vi "Read Device Identification.vi"(8 "error in (no error)":errorcluster, 9 "object ID":u8, 10 "device ID category":T1(ring), 11 "Modbus master in":refnum<class "Modbus Master.lvclass">) -> (0 "error out":errorcluster, 2 "objects":cluster{"object ID":u8, "value":string}[](array[cluster]) {"object ID" format="%x"}, 3 "Modbus master out":refnum<class "Modbus Master.lvclass">)   [LabVIEW 2017, in "Modbus Master.lvclass"]
doc: "Returns the device identification of a Modbus slave. Device identification consists of data elements called objects. Each object has an identification number and stores Modbus slave information."
uses:
  <vilib>/Modbus/master/Modbus Master.lvclass
  C:/builds/penguin/iak/lvdsc/trunk/17.0/lv/vi.lib/Modbus/subvis/Modbus API/Modbus API.lvclass
  <vilib>/Modbus/subvis/Modbus API/Modbus API.lvclass/Modbus API.ctl
  <vilib>/Modbus/master/Modbus Master.lvclass/Modbus Master.ctl
  <vilib>/Modbus/subvis/Protocol/Interfaces/Network Master/Network Master.lvclass
  C:/builds/penguin/iak/lvdsc/trunk/17.0/lv/vi.lib/Modbus/subvis/Protocol/Interfaces/Network Protocol/Network Protocol.lvclass
  <vilib>/Modbus/subvis/Transmission Data Unit (ADU)/Transmission Data Unit/Transmission Data Unit.lvclass
  <vilib>/Modbus/subvis/Modbus API/Modbus API.lvclass
  <vilib>/Modbus/subvis/Data and Functions/Master Function Definition/Master Function Definition.lvlib
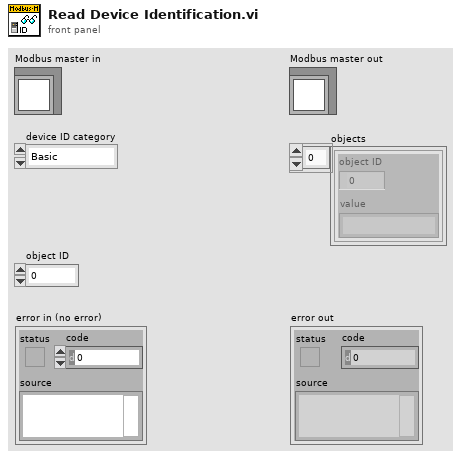
[diagram p1: front panel]
types:
  T1 = enum8{"Basic", "Regular", "Extended", "Specific"}
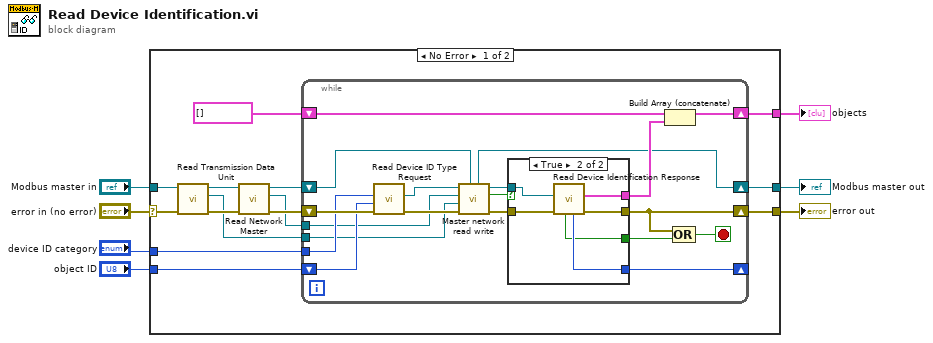
[diagram p0: block diagram]
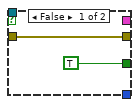
[diagram p2: hidden frame]
diagram:
  n1 = case shown="No Error" "error in (no error)" {
    selector: "error in (no error)" -> [w8 w50]
    tunnel: "Modbus master in" -> [w9 w49]
    tunnel: [w16 w49] -> w5
    tunnel: [w17 w50] -> w4
    tunnel: "device ID category" -> [w21 _]
    tunnel: "object ID" -> [w20 _]
    tunnel: [w19 _] -> w2
    frame No Error {
      n2 = call <vilib>:"Read Transmission Data Unit.vi"("error in (no error)"=w8, "Modbus instance in"=w9) -> ("error out"=w12:errorcluster, "transmission data unit"=w11:refnum<class "Transmission Data Unit.lvclass">, "Modbus instance out"=w13:refnum<class "Modbus Master.lvclass">)  [unwired: 7 in]
      n3 = call <vilib>:"Read Network Master.vi"("error in (no error)"=w12, "Modbus master in"=w13) -> ("error out"=w15:errorcluster, "network master"=w10:refnum<class "Network Master.lvclass">, "Modbus master out"=w14:refnum<class "Modbus Master.lvclass">)  [unwired: 7 in]
      n4 = while {
        tunnel: w21 -> [w39]
        shift-right: [w36] -> w17
        shift-left: w15 -> [w40]
        shift-right: [w35] -> w19
        shift-left: cluster{"object ID":u8, "value":string}[] [] -> [w34]
        shift-right: [w33] -> _
        shift-left: w20 -> [w38]
        shift-right: [w26] -> w16
        shift-left: w14 -> [w25]
        tunnel: w11 -> [w24]
        tunnel: w10 -> [w23]
        stop <- w37 stop-if-true
        n5 = call <vilib>:"Read Device ID Type Request.vi"("error in (no error)"=w40, "object ID"=w38, "read device ID code"=w39) -> ("error out"=w27:errorcluster, "Modbus data unit out"=w28:refnum<class "Modbus Data Unit (PDU).lvclass">)  [unwired: 7 in]
        n6 = call <vilib>:"Master network read write.vi"("Modbus master in"=w25, "error in (no error)"=w27, "transmission data unit in"=w24, "network master in"=w23, "Modbus data unit in"=w28) -> ("error out"=w30:errorcluster, "PDU valid?"=w22:bool, "Modbus data unit out"=w29:refnum<class "Modbus Data Unit (PDU).lvclass">, "Modbus master out"=w26:refnum<class "Modbus Master.lvclass">)  [unwired: 3 in]
        n7 = case shown="True" w22 {
          tunnel: [w42 w48] -> w36
          tunnel: [_ w47] -> w33
          tunnel: [TRUE ("done?") w46] -> w32
          tunnel: [_ w45] -> w31
          tunnel: w30 -> [w42 w44]
          tunnel: w29 -> [_ w43]
          frame False {
          }
          frame True {
            n8 = call <vilib>:"Read Device Identification Response.vi"("error in (no error)"=w44, "Modbus data unit in"=w43) -> ("error out"=w48:errorcluster, "objects"=w45:cluster{"object ID":u8, "value":string}[], "next object ID"=w47:u8, "done?"=w46:bool)  [unwired: 5 in, 1 out]
          }
        }
        n9 = Build Array (concatenate)(w34, w31) -> (w35:cluster{"object ID":u8, "value":string}[])
        n10 = Compound Arithmetic op=OR(w36, w32) -> (w37:bool)
      }
    }
    frame Error {
    }
  }
  "error out" <- w4
  "Modbus master out" <- w5
  "objects" <- w2
